vi "SMD7615 UDP Init.vi"(8 "error in (no error)":errorcluster, 10 "IP":string="192.168.1.30", 11 "connection ID in":refnum<k16>) -> (0 "error out":errorcluster, 3 "connection ID out":refnum<k16>)   [LabVIEW 2016, in "SMD-7615.lvlib" / "eSCL.lvlib"]
uses:
  eSCL.lvlib
panel:
  out "Status 2":string
  out "Status":string
  out "Model & Revision":string
  out "RLR":string
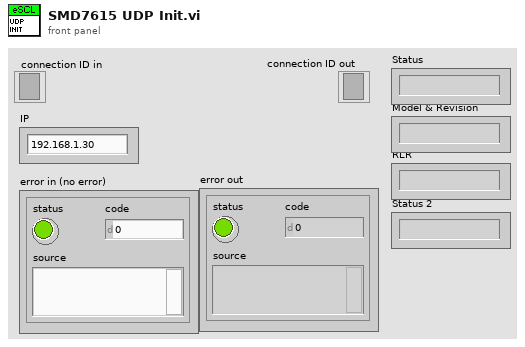
[diagram p1: front panel]
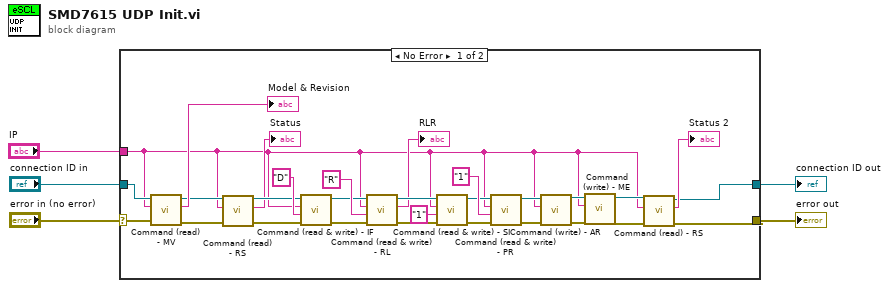
[diagram p0: block diagram]
diagram:
  n1 = case shown="No Error" "error in (no error)" {
    selector: "error in (no error)" -> [w15 w35]
    tunnel: "connection ID in" -> [w14 w36]
    tunnel: [w7 w36] -> w3
    tunnel: [w6 w35] -> w2
    tunnel: "IP" -> [w8 _]
    frame No Error {
      n2 = call "Command (read) - MV.vi"("error in (no error)"=w15, "IP"=w8, "connection ID in"=w14) -> ("error out"=w18:errorcluster, "Model & Revision"=→"Model & Revision":string, "connection ID out"=w17:refnum<k16>)  [unwired: 6 in]
      n3 = call "Command (read) - RS.vi"("error in (no error)"=w18, "IP"=w8, "connection ID in"=w17) -> ("error out"=w21:errorcluster, "Status"=→"Status":string, "connection ID out"=w20:refnum<k16>)  [unwired: 6 in]
      n4 = call "Command (read & write) - IF.vi"("error in (no error)"=w21, "Format"="D", "IP"=w8, "connection ID in"=w20) -> ("error out"=w24:errorcluster, "connection ID out"=w23:refnum<k16>)  [unwired: 6 in]
      n5 = call "Command (read & write) - RL.vi"("error in (no error)"=w24, "Register"="R", "IP"=w8, "connection ID in"=w23) -> ("error out"=w27:errorcluster, "Register Value"=→"RLR":string, "connection ID out"=w28:refnum<k16>)  [unwired: 5 in]
      n6 = call "Command (read & write) - SI.vi"("error in (no error)"=w27, "Input Usage State"="1", "IP"=w8, "connection ID in"=w28) -> ("error out"=w31:errorcluster, "connection ID out"=w30:refnum<k16>)  [unwired: 5 in, 1 out]
      n7 = call "Command (read & write) - PR.vi"("error in (no error)"=w31, "Protocol Setting"="1", "IP"=w8, "connection ID in"=w30) -> ("error out"=w34:errorcluster, "connection ID out"=w33:refnum<k16>)  [unwired: 5 in, 1 out]
      n8 = call "Command (write) - AR.vi"("error in (no error)"=w34, "IP"=w8, "connection ID in"=w33) -> ("error out"=w13:errorcluster, "connection ID out"=w12:refnum<k16>)  [unwired: 7 in]
      n9 = call "Command (write) - ME.vi"("error in (no error)"=w13, "IP"=w8, "connection ID in"=w12) -> ("error out"=w11:errorcluster, "connection ID out"=w10:refnum<k16>)  [unwired: 7 in]
      n10 = call "Command (read) - RS.vi"("error in (no error)"=w11, "IP"=w8, "connection ID in"=w10) -> ("error out"=w6:errorcluster, "Status"=→"Status 2":string, "connection ID out"=w7:refnum<k16>)  [unwired: 6 in]
    }
    frame Error {
    }
  }
  "connection ID out" <- w3
  "error out" <- w2
